vi "Get Angle Error.vi"(10 "Goal Angles":T3, 11 "Real Angles":T4) -> (2 "Motor Power":T1, 3 "Angle Error":T2)   [LabVIEW 2018]
uses:
  <vilib>/Rock Robotics/Network Tables/NT Write Number.vi
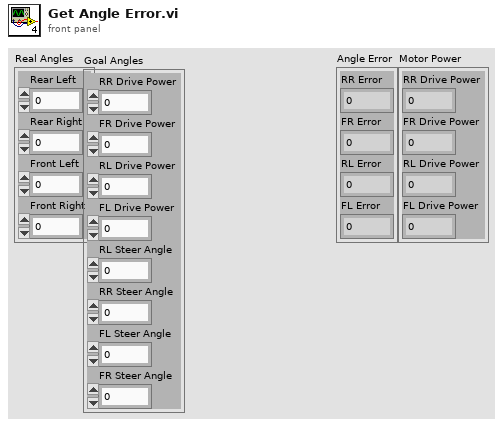
[diagram p1: front panel]
types:
  T1 = cluster{"RR Drive Power":dbl, "FR Drive Power":dbl, "RL Drive Power":dbl, "FL Drive Power":dbl}
  T2 = cluster{"RR Error":dbl, "FR Error":dbl, "RL Error":dbl, "FL Error":dbl}
  T3 = cluster{"RR Drive Power":dbl, "FR Drive Power":dbl, "RL Drive Power":dbl, "FL Drive Power":dbl, "RL Steer Angle":dbl, "RR Steer Angle":dbl, "FL Steer Angle":dbl, "FR Steer Angle":dbl}
  T4 = cluster{"Rear Left":dbl, "Rear Right":dbl, "Front Left":dbl, "Front Right":dbl}
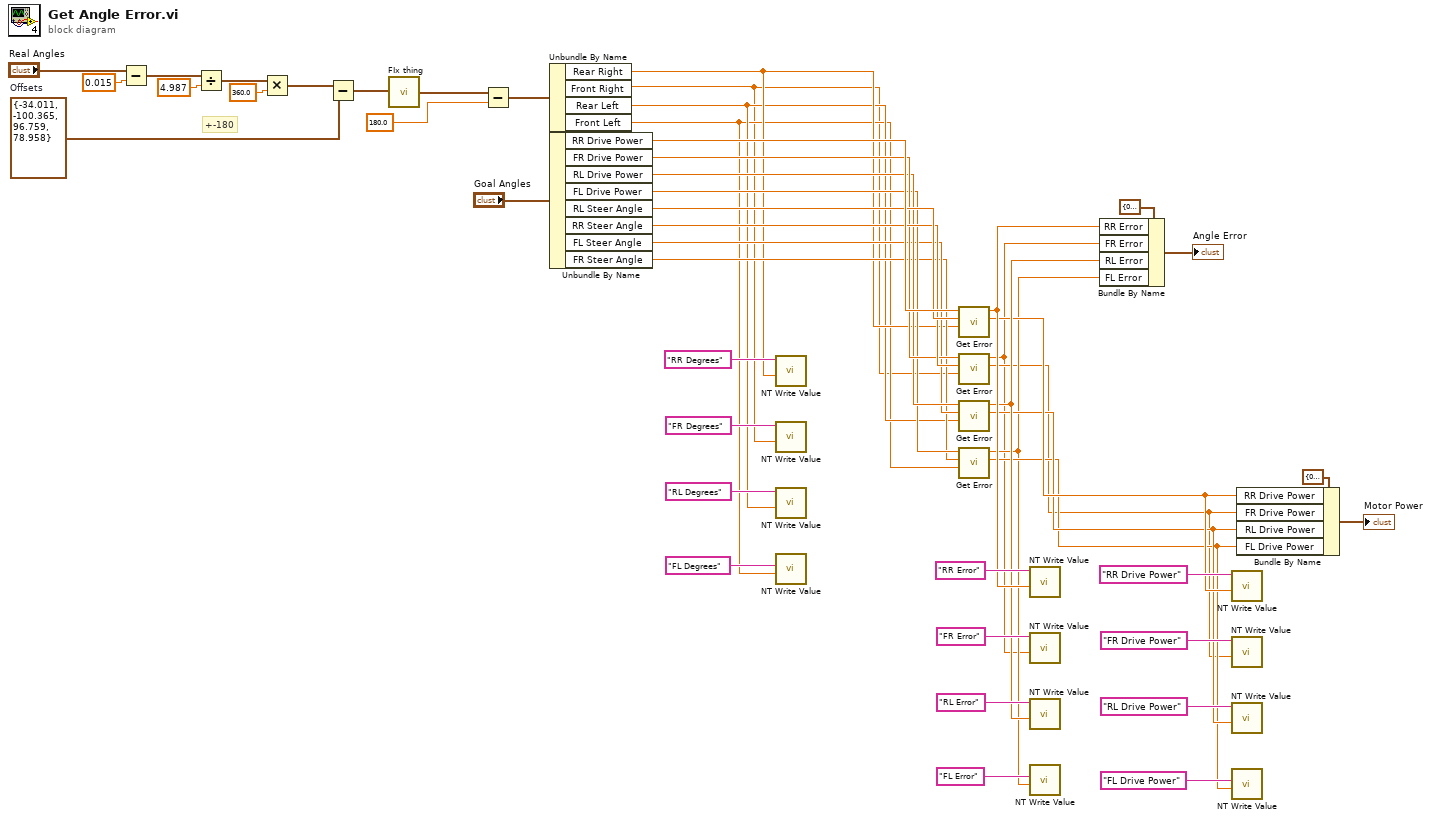
[diagram p0: block diagram]
diagram:
  w23 = T4 {"Rear Left"=-34.011, "Rear Right"=-100.365, "Front Left"=96.759, "Front Right"=78.958}  # Offsets
  # "+-180"
  n1 = Subtract(x="Real Angles", y=0.015) -> (x-y=w47:T4)
  n2 = Divide(x=w47, y=4.987) -> (x/y=w45:T4)
  n3 = Multiply(x=w45, y=360.0) -> (x*y=w43:T4)
  n4 = Subtract(x=w43, y=w23) -> (x-y=w22:T4)
  n5 = call "FIx thing.vi"("Input"=w22) -> ("Output"=w21:T4)
  n6 = Subtract(x=w21, y=180.0) -> (x-y=w25:T4)
  n7 = Unbundle By Name(w25) -> ("Rear Right"=w20:dbl, "Front Right"=w1:dbl, "Rear Left"=w19:dbl, "Front Left"=w2:dbl)
  n8 = Unbundle By Name("Goal Angles") -> ("RR Drive Power"=w41:dbl, "FR Drive Power"=w38:dbl, "RL Drive Power"=w37:dbl, "FL Drive Power"=w36:dbl, "RL Steer Angle"=w40:dbl, "RR Steer Angle"=w39:dbl, "FL Steer Angle"=w35:dbl, "FR Steer Angle"=w34:dbl)
  n9 = call-poly <vilib>:"NT Write Value.vi"("Numeric"=w20, "Name"="RR Degrees") -> ()  [unwired: 9 in, 1 out]
  n10 = call-poly <vilib>:"NT Write Value.vi"("Numeric"=w1, "Name"="FR Degrees") -> ()  [unwired: 9 in, 1 out]
  n11 = call-poly <vilib>:"NT Write Value.vi"("Numeric"=w19, "Name"="RL Degrees") -> ()  [unwired: 9 in, 1 out]
  n12 = call-poly <vilib>:"NT Write Value.vi"("Numeric"=w2, "Name"="FL Degrees") -> ()  [unwired: 9 in, 1 out]
  n13 = call "Get Error.vi"("Actual Angle"=w20, "Desired Angle"=w40, "Motor Power"=w41) -> ("Motor Power"=w8:dbl, "Angle Error"=w14:dbl)  [unwired: 7 in]
  n14 = call "Get Error.vi"("Actual Angle"=w1, "Desired Angle"=w39, "Motor Power"=w38) -> ("Motor Power"=w4:dbl, "Angle Error"=w3:dbl)  [unwired: 7 in]
  n15 = call "Get Error.vi"("Actual Angle"=w19, "Desired Angle"=w35, "Motor Power"=w37) -> ("Motor Power"=w7:dbl, "Angle Error"=w13:dbl)  [unwired: 7 in]
  n16 = call "Get Error.vi"("Actual Angle"=w2, "Desired Angle"=w34, "Motor Power"=w36) -> ("Motor Power"=w6:dbl, "Angle Error"=w5:dbl)  [unwired: 7 in]
  n17 = call-poly <vilib>:"NT Write Value.vi"("Numeric"=w14, "Name"="RR Error") -> ()  [unwired: 9 in, 1 out]
  n18 = call-poly <vilib>:"NT Write Value.vi"("Numeric"=w3, "Name"="FR Error") -> ()  [unwired: 9 in, 1 out]
  n19 = call-poly <vilib>:"NT Write Value.vi"("Numeric"=w13, "Name"="RL Error") -> ()  [unwired: 9 in, 1 out]
  n20 = call-poly <vilib>:"NT Write Value.vi"("Numeric"=w5, "Name"="FL Error") -> ()  [unwired: 9 in, 1 out]
  n21 = Bundle By Name(cluster=T2 {"RR Error"=0.0, "FR Error"=0.0, "RL Error"=0.0, "FL Error"=0.0} ("Angle Error 2"), "RR Error"=w14, "FR Error"=w3, "RL Error"=w13, "FL Error"=w5) -> (→"Angle Error":T2)
  n22 = call-poly <vilib>:"NT Write Value.vi"("Numeric"=w8, "Name"="RR Drive Power") -> ()  [unwired: 9 in, 1 out]
  n23 = call-poly <vilib>:"NT Write Value.vi"("Numeric"=w4, "Name"="FR Drive Power") -> ()  [unwired: 9 in, 1 out]
  n24 = call-poly <vilib>:"NT Write Value.vi"("Numeric"=w7, "Name"="RL Drive Power") -> ()  [unwired: 9 in, 1 out]
  n25 = call-poly <vilib>:"NT Write Value.vi"("Numeric"=w6, "Name"="FL Drive Power") -> ()  [unwired: 9 in, 1 out]
  n26 = Bundle By Name(cluster=T1 {"RR Drive Power"=0.0, "FR Drive Power"=0.0, "RL Drive Power"=0.0, "FL Drive Power"=0.0} ("Motor Power 2"), "RR Drive Power"=w8, "FR Drive Power"=w4, "RL Drive Power"=w7, "FL Drive Power"=w6) -> (→"Motor Power":T1)
